vi "pulse_from memory tester.vi"() -> ()   [LabVIEW 2021]
uses:
  CTL/emitter params.ctl
  CTL/mode_type.ctl
  pdw.ctl
  <vilib>/addons/Modulation/Analog/controls/Complex Data Waveform.ctl
  <instrlib>/_niInstr/DSP/v1/Shared/Public/IQ Data.ctl
  <vilib>/addons/Modulation/Analog/support/Validators/mod_Fractional Resample Validate.vi
  <vilib>/addons/Modulation/Analog/support/Validators/mod_Check Flush State.vi
  <vilib>/addons/Modulation/Analog/support/mod_FractionalResampler.vi
  <vilib>/addons/Modulation/Analog/support/mod_Integer Rate Interpolation.vi
  <vilib>/addons/Modulation/Analog/support/mod_Set Error Source.vi
  <vilib>/addons/Modulation/Analog/support/Validators/mod_Validate Complex Waveform.vi
  <vilib>/addons/Modulation/Analog/support/mod_PerformResampling.vi
  <vilib>/addons/Modulation/Analog/support/Validators/mod_WFErrorHandler.vi
  <vilib>/sound2/lvsound2.llb/Sound File Read Open.vi
  <vilib>/sound2/lvsound2.llb/Sound File Read (DBL).vi
  <vilib>/Utility/error.llb/Error Cluster From Error Code.vi
  <vilib>/addons/Modulation/Analog/support/mod_Resampling Factors.vi
  <vilib>/addons/Modulation/Analog/support/mod_ResamplingFilter.vi
  <vilib>/addons/Modulation/Analog/support/mod_Generate Integer Interpolation Filter.vi
  <instrlib>/_niInstr/DSP/v1/FPGA/Public/Sub VIs/Data Conversion/IQ to U32 - 1 spc - S18.1.vi
  <vilib>/measure/maspectr.llb/FFT Power Spectrum and PSD for 1 Chan (CDB).vi
  <instrlib>/_niInstr/DSP/v1/FPGA/Public/Sub VIs/Data Conversion/U32 to IQ - N spc - S18.1.vi
  <vilib>/Analysis/NI_AALPro.lvlib
  <vilib>/measure/NI_MAPro.lvlib
  <instrlib>/_niInstr/Basic Elements/v1/FPGA/niInstr Basic Elements v1 FPGA.lvlib
  <vilib>/addons/Modulation/niAMT.lvlib
  <instrlib>/_niInstr/DSP/v1/Shared/niInstr DSP v1 Shared.lvlib
  <instrlib>/_niInstr/DSP/v1/FPGA/niInstr DSP v1 FPGA.lvlib
panel:
  in  "random bar":dbl
  out "start index":u16[](array[numeric])
  out "length":u16[](array[numeric])
  out "memory data":u32[](array[numeric])
  out "memory status 2":dbl[](graph)
  out "memory status":u32[](graph)
  out "Numeric":i32
  in  "num file":i32
  in  "IQ files":path[](array[path])=[path "C:/Users/PXIe8108_Demo/Documents/CHAIM DATA/chaim/5785_sync_for_elbit/tx_pulse/pulse Tx Folder_lv_21/EMEA_ADG_EW_Multi_Emitter_Scenarios/data/comb.wav"]
  out "D phase to Dt":dbl[](graph)
  out "output valid":i16[](graph)
  out "PDW in":T1={"PW"=60000, "frequency shift"=0.004999999999999005, "amp"=0.31623077392578125, "mode type"=enum."LFM", "mode depth"=234562481, "mode filter"=0, "phase shift"=0.0, "pulse shape filter"=0}
  out "free DDS":i16[](graph)
  out "Power Spectrum / PSD":cluster{"f0":dbl, "df":dbl, "magnitude":dbl[]}[](graph)
  out "amp out":dbl[](graph)
  out "phase out":dbl[](graph)
  in  "num of sampels for test":i32=30000 format="%.0p"
  out "I data":dbl[](graph)
  in  "emmiter":T3[](array[typedef])=[{"f set"=[1000000.0], "hop rate (Hz)"=1000.0, "d.c."=0.1, "amp (dB)"=-10.0, "mod type"=enum."from memory 1", "mod depth"=0.0, "DOA"=0.0, "t start"=0.0, "t end"=3.0}] {"t end" format="%#_3p"; "t start" format="%#_3p"; "DOA" format="%#_3p"; "mod depth" format="%.0p"}
  in  "Fs":i32=200000000 format="%#.3p"
  # "mode type:\n0- cw\n3-lfm\n4- bpsk\n5-qpsk"
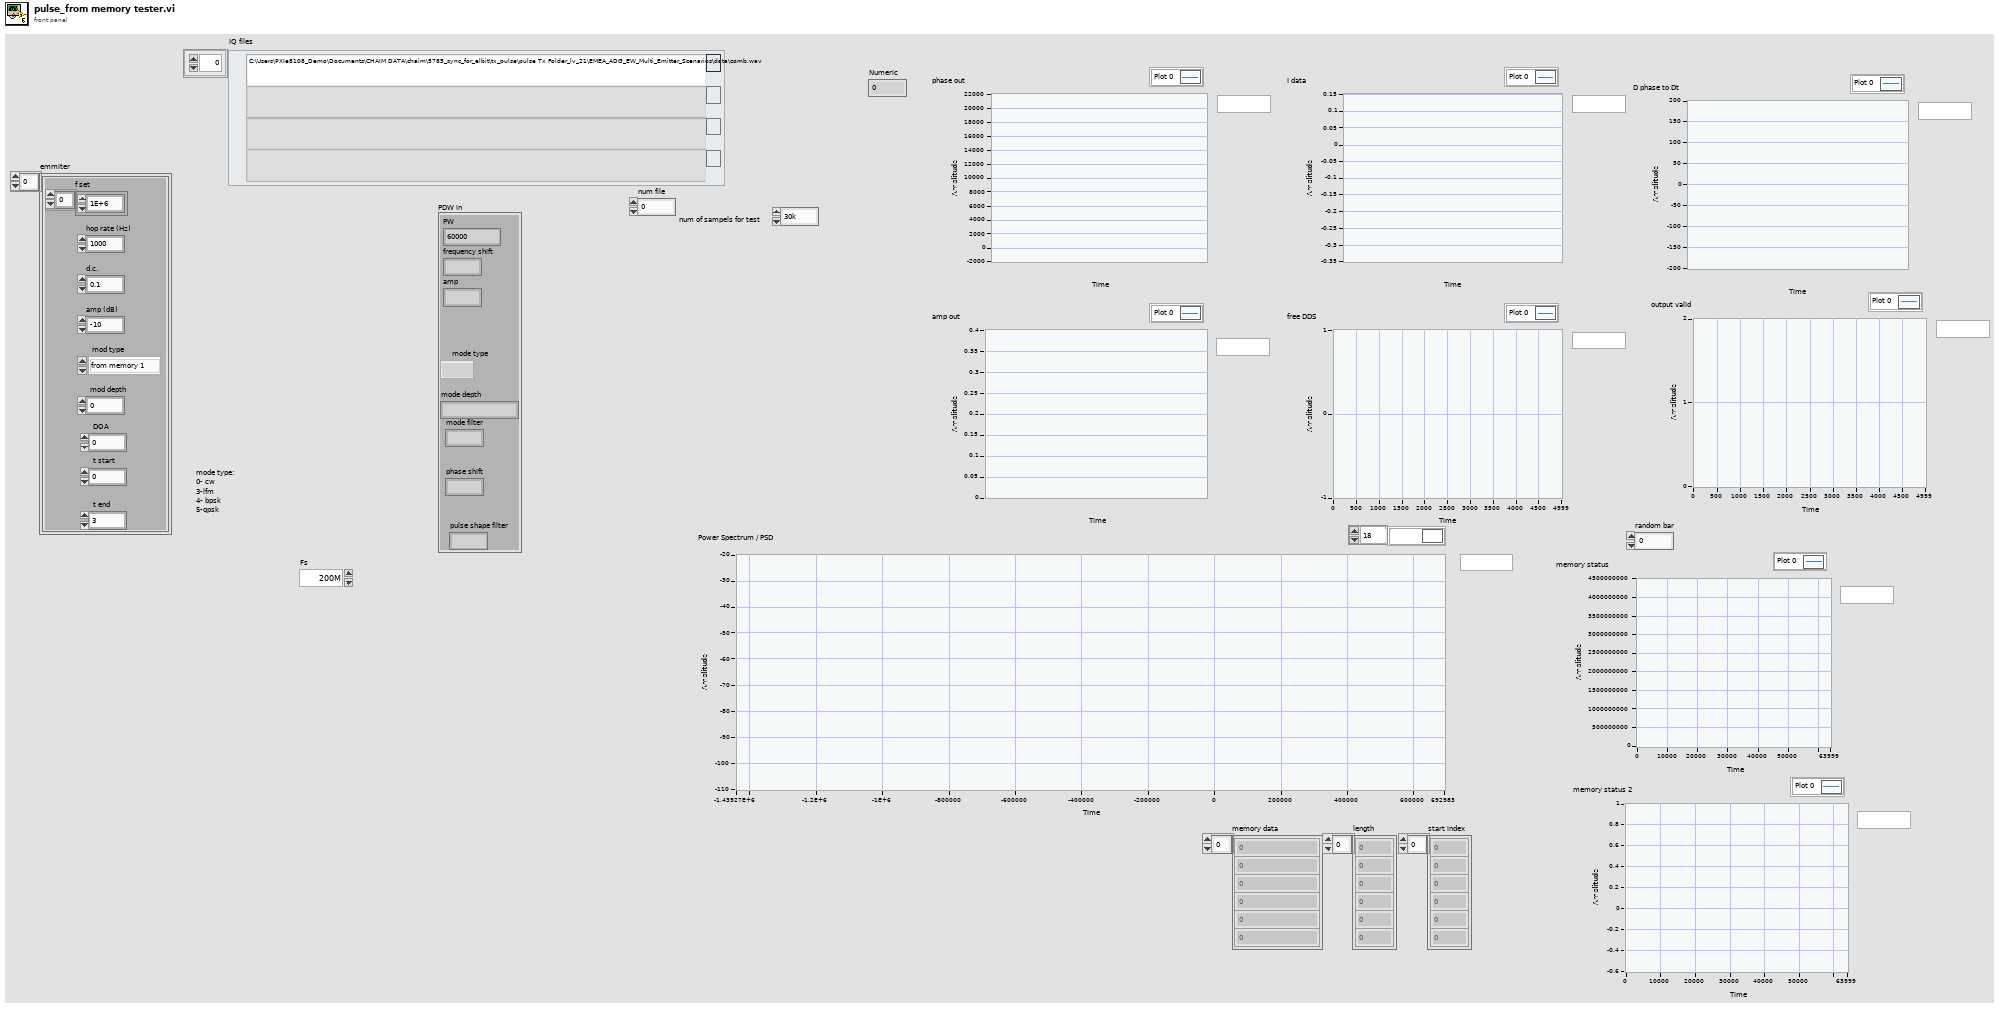
[diagram p1: front panel]
types:
  T1 = typedef "pdw.ctl" = cluster{"PW":u32, "frequency shift":fxp<+/-,48,0>, "amp":fxp<+/-,18,1>, "mode type":T2, "mode depth":u32, "mode filter":u8, "phase shift":fxp<+/-,16,1>, "pulse shape filter":u8}
  T2 = typedef "mode_type.ctl" = enum8{"CW", "from memory 1", "NC - cw", "LFM", "BPSK", "QPSK"}
  T3 = typedef "emitter params.ctl" = cluster{"f set":dbl[], "hop rate (Hz)":dbl, "d.c.":dbl, "amp (dB)":dbl, "mod type":T2, "mod depth":dbl, "DOA":dbl, "t start":dbl, "t end":dbl}
  T4 = typedef "niAMT.lvlib/Complex Data Waveform.ctl" = cluster{"t0":dbl, "dt":dbl, "Y":cdb[]}
  T5 = typedef "niInstr DSP v1 Shared.lvlib/IQ Data.ctl" = cluster{"I":fxp<+/-,18,1>, "Q":fxp<+/-,18,1>, "overflow":bool}
  T6 = typedef "Sound File Refnum.ctl" = refnum<file>
  T7 = typedef "PDW_lv2.ctl" = cluster{"t start":dbl, "frequency (Hz)":dbl, "duration (sec)":dbl, "mod type":T2, "mod depth":dbl, "phase (rad)":dbl[], "amp (lin)":dbl[]}
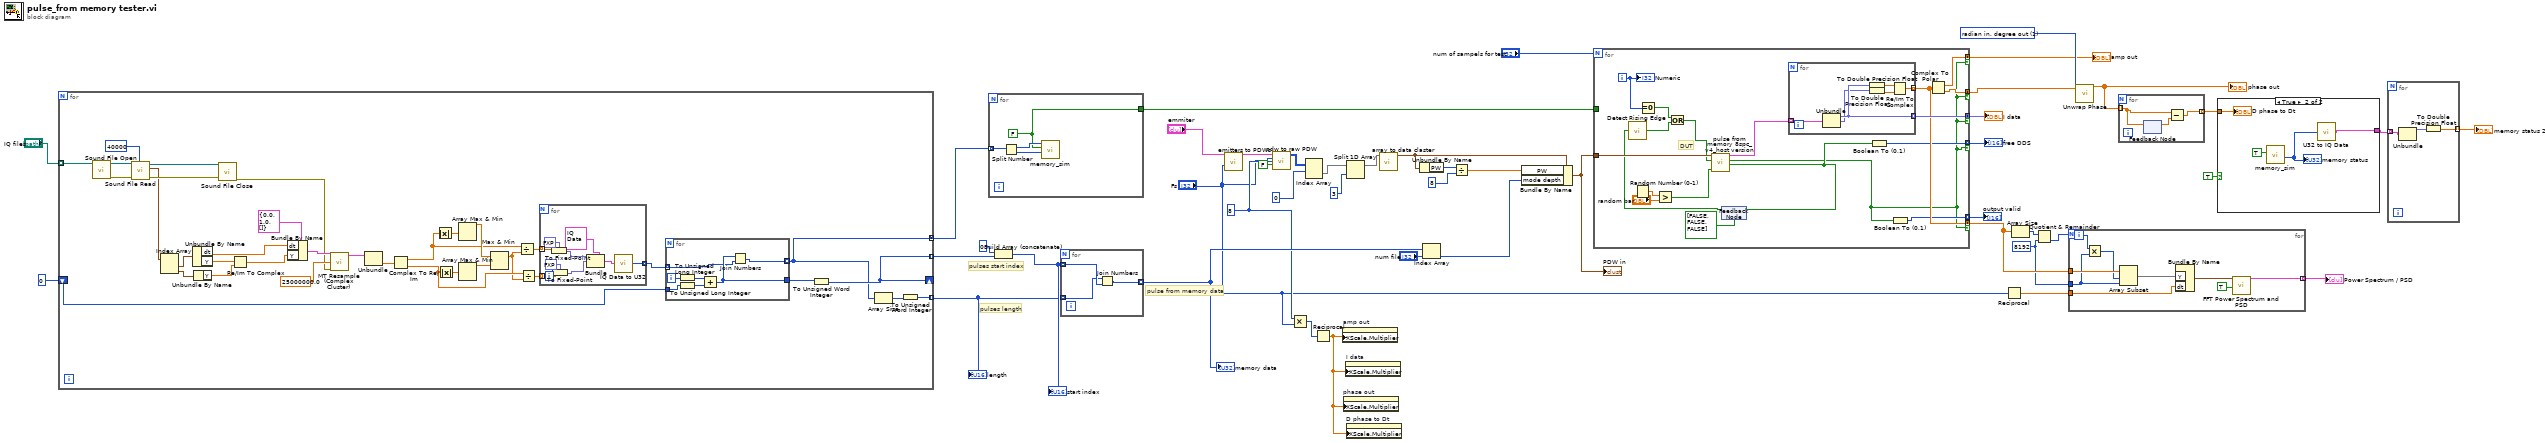
[diagram p0: block diagram]
diagram:
  w4 = 8 ("SPC")
  w35 = 8192 ("length")
  w44 = 1 items=["radian in, radian out", "radian in, degree out", "degree in, degree out", "degree in, radian out"] ("phase unit")
  # "pulse from memory data"
  # "pulses start index"
  # "pulses length"
  n1 = for {
    shift-right: [w53] -> _
    shift-left: u16 0 -> [w55]
    tunnel: [w48] -> w18 mode=concatenating
    tunnel: [w51] -> w20 mode=indexing
    tunnel: [w53] -> w19 mode=indexing
    tunnel: "IQ files" -> [w50] mode=indexing
    n2 = call-poly <vilib>:"Sound File Open.vi"("path"=w50) -> ("error out"=w78:errorcluster, "sound file refnum"=w81:T6)  [unwired: 9 in]
    n3 = call-poly <vilib>:"Sound File Read.vi"("number of samples/ch (-1: all)"=40000, "error in (no error)"=w78, "sound file refnum"=w81) -> ("error out"=w77:errorcluster, "data"=w76:waveform(dbl)[], "sound file refnum out"=w80:T6)  [unwired: 4 in, 2 out]
    n4 = Index Array(array=w76) -> (element #1=w75:waveform(dbl), element #2=w74:waveform(dbl))  [unwired: 2 in]
    n5 = Unbundle By Name(w75) -> ("dt"=w70:dbl, "Y"=w73:dbl[])
    n6 = Unbundle By Name(w74) -> ("Y"=w72:dbl[])
    n7 = call <vilib>:"Sound File Close.vi"("error in (no error)"=w77, "sound file refnum"=w80) -> ("error out"=w60:errorcluster)  [unwired: 9 in]
    n8 = Re/Im To Complex(1:w72, 2:w73) -> (0:w69:cdb[])
    n9 = Bundle By Name(cluster=T4 {"t0"=0.0, "dt"=1.0, "Y"=[]} ("input complex waveform"), "dt"=w70, "Y"=w69) -> (w68:T4)
    n10 = call <vilib>:"MT Resample (Complex Cluster).vi"("input complex waveform"=w68, "desired sample rate (Hz)"=25000000.0, "error in (no error)"=w60) -> ("output complex waveform"=w58:T4)  [unwired: 11 in, 1 out]
    n11 = Unbundle(w58) -> ("Y"=w66:cdb[])  [unwired: 2 out]
    n12 = Complex To Re/Im(x + iy=w66) -> (x=w49:dbl[], y=w61:dbl[])
    n13 = Absolute Value(x=w49) -> (abs(x)=w63:dbl[])
    n14 = Absolute Value(x=w61) -> (abs(x)=w62:dbl[])
    n15 = Array Max & Min(array=w63) -> (max value=w64:dbl)  [unwired: 3 out]
    n16 = Array Max & Min(array=w62) -> (max value=w65:dbl)  [unwired: 3 out]
    n17 = Max & Min(x=w64, y=w65) -> (max(x,y)=w59:dbl)  [unwired: 1 out]
    n18 = Divide(x=w49, y=w59) -> (x/y=w57:dbl[])
    n19 = Divide(x=w61, y=w59) -> (x/y=w47:dbl[])
    n20 = for {
      tunnel: w47 -> [w88] mode=indexing
      tunnel: w57 -> [w85] mode=indexing
      tunnel: [w82] -> w56 mode=indexing
      n21 = To Fixed-Point(fixed-point type=fxp<+/-,18,1> 0.0 ("I"), number=w85) -> (fixed-point=w84:fxp<+/-,18,1>)
      n22 = To Fixed-Point(fixed-point type=fxp<+/-,18,1> 0.0 ("I"), number=w88) -> (fixed-point=w89:fxp<+/-,18,1>)
      n23 = Bundle(cluster=T5 {"I"=0.0, "Q"=0.0, "overflow"=FALSE} ("IQ data"), "I"=w84, "Q"=w89) -> (w83:T5)  [unwired: 1 in]
      n24 = call-poly <instrlib>:"IQ Data to U32.vi"("IQ data"=w83) -> ("U32 data"=w82:u32)  [unwired: 13 in, 1 out]
    }
    n25 = for {
      tunnel: [w97] -> w48 mode=indexing
      tunnel: [w96] -> w54
      tunnel: w55 -> [w92]
      tunnel: w56 -> [w95] mode=indexing
      i -> [w94]
      n26 = To Unsigned Long Integer(number=w94) -> (unsigned 32bit integer=w93:u32)
      n27 = To Unsigned Long Integer(number=w92) -> (unsigned 32bit integer=w91:u32)
      n28 = Add(x=w93, y=w91) -> (x+y=w96:u32)
      n29 = Join Numbers(hi=w96, lo=w95) -> ((hi.lo)=w97:u64)
    }
    n30 = To Unsigned Word Integer(number=w54) -> (unsigned 16bit integer=w53:u16)
    n31 = Array Size(array=w48) -> (size(s)=w52:i32)
    n32 = To Unsigned Word Integer(number=w52) -> (unsigned 16bit integer=w51:u16)
  }
  "length" <- w20
  n33 = for {
    tunnel: w18 -> [w101] mode=indexing
    tunnel: [w98] -> w1
    w98 = FALSE ("t-read;fwrite")
    n34 = Split Number(x=w101) -> (hi(x)=w100:u32, lo(x)=w99:u32)
    n35 = call "memory_sim.vi"("data in"=w99, "t-read;fwrite"=w98, "index"=w100) -> ()  [unwired: 7 in, 2 out]
  }
  n36 = Build Array (concatenate)(u16 0, w19) -> (w22:u16[])
  "start index" <- w22
  n37 = for {
    tunnel: w22 -> [w104] mode=indexing
    tunnel: w20 -> [w103] mode=indexing
    tunnel: [w102] -> w17 mode=indexing
    n38 = Join Numbers(hi=w103, lo=w104) -> ((hi.lo)=w102:u32)
  }
  "memory data" <- w17
  n39 = call "emitters to PDWs.vi"("emmiter"="emmiter", "center frequency (Hz)"="Fs") -> ("sorted array"=w41:T7[])  [unwired: 11 in, 2 out]
  n40 = call "pdw to raw PDW.vi"("PDWs"=w41, "Fs fpGa"="Fs", "SPC"=w4, "gen for DF"=FALSE) -> ("Array"=w29:u64[][])  [unwired: 9 in, 2 out]
  n41 = Multiply(x=w4, y="Fs") -> (x*y=w2:i32)
  n42 = Index Array(array=w29, index (row)=0) -> (element=w26:u64[])  [unwired: 1 in]
  n43 = Reciprocal(x=w2) -> (1/x=w5:dbl)
  n44 = property on="amp out" class="WFGraph (strict)"("XScale.Multiplier"=w5) -> ()  [unwired: 2 in, 2 out]
  n45 = property on="phase out" class="WFGraph (strict)"("XScale.Multiplier"=w5) -> ()  [unwired: 2 in, 2 out]
  n46 = property on="I data" class="WFGraph (strict)"("XScale.Multiplier"=w5) -> ()  [unwired: 2 in, 2 out]
  n47 = property on="D phase to Dt" class="WFGraph (strict)"("XScale.Multiplier"=w5) -> ()  [unwired: 2 in, 2 out]
  n48 = Split 1D Array(array=w26, index=3) -> (first subarray=w24:u64[])  [unwired: 1 out]
  n49 = call "array to data claster.vi"("Array"=w24) -> ("Cluster"=w9:T1)  [unwired: 10 in]
  n50 = Unbundle By Name(w9) -> ("PW"=w8:u32)
  n51 = Index Array(array=w17, index="num file") -> (element=w15:u32)
  n52 = Divide(x=w8, y=u32 8) -> (x/y=w6:dbl)
  n53 = Bundle By Name(cluster=w9, "PW"=w6, "mode depth"=w15) -> (w10:T1)
  "PDW in" <- w10
  n54 = for {
    N: "num of sampels for test" -> [_]
    tunnel: [w122] -> w46 mode=concatenating if=w110
    tunnel: [w119] -> w45 mode=concatenating if=w110
    tunnel: [w120] -> w43 mode=concatenating if=w110
    tunnel: w10 -> [w121]
    tunnel: [w118] -> w39 mode=concatenating if=w110
    tunnel: [w117] -> w37 mode=indexing if=w110
    tunnel: [w116] -> w32 mode=indexing
    tunnel: w1 -> [_]
    i -> [w108]
    # "DUT"
    n55 = Random Number (0-1)() -> (number: 0 to 1=w113:dbl)
    n56 = Equal To 0?(x=w108) -> (x = 0?=w107:bool)
    n57 = Greater?(x=w113, y="random bar") -> (0:w111:bool)
    n58 = feedback #1(bool[] [FALSE, FALSE, FALSE]) -> (w115:bool)
    n59 = call <instrlib>:"Detect Rising Edge.vi"("signal"=w115) -> ("edge detected"=w106:bool)  [unwired: 14 in]
    n60 = Or(x=w107, y=w106) -> (x .or. y?=w105:bool)
    n61 = call "pulse from memory 8spc_v4_host version.vi"("run"=w111, "start this pulse"=w105, "PDW"=w121) -> ("free DDS"=w114:bool, "output valid"=w110:bool, "IQ_out"=w123:T5[])  [unwired: 6 in]
    n62 = feedback-in #1(w114) -> ()
    n63 = for {
      tunnel: w123 -> [w129] mode=indexing
      tunnel: [w128] -> w122 mode=indexing
      tunnel: [w126] -> w118 mode=indexing
      n64 = Unbundle(w129) -> ("I"=w128:fxp<+/-,18,1>, "Q"=w127:fxp<+/-,18,1>)  [unwired: 1 out]
      n65 = To Double Precision Float(number=w128) -> (double precision float=w125:dbl)
      n66 = To Double Precision Float(number=w127) -> (double precision float=w124:dbl)
      n67 = Re/Im To Complex(1:w124, 2:w125) -> (0:w126:cdb)
    }
    n68 = Boolean To (0,1)(Boolean=w114) -> (0, 1=w117:i16)
    n69 = Boolean To (0,1)(Boolean=w110) -> (0, 1=w116:i16)
    n70 = Complex To Polar(r * e^(i*theta)=w118) -> (r=w120:dbl[], theta=w119:dbl[])
    "Numeric" <- w108
  }
  "I data" <- w46
  "amp out" <- w43
  "free DDS" <- w37
  "output valid" <- w32
  n71 = Reciprocal(x="Fs") -> (1/x=w40:dbl)
  n72 = Array Size(array=w39) -> (size(s)=w36:i32)
  n73 = Quotient & Remainder(x=w36, y=w35) -> (floor(x/y)=w34:i32)  [unwired: 1 out]
  n74 = for {
    N: w34 -> [_]
    tunnel: w39 -> [w135]
    tunnel: w40 -> [w134]
    tunnel: w35 -> [w133]
    tunnel: [w131] -> w33 mode=indexing
    i -> [w130]
    n75 = Multiply(x=w130, y=w133) -> (x*y=w132:i32)
    n76 = Array Subset(array=w135, index=w132, length=w133) -> (w136:cdb[])
    n77 = Bundle By Name("Y"=w136, "dt"=w134) -> (w138:waveform(cdb))  [unwired: 1 in]
    n78 = call-poly <vilib>:"FFT Power Spectrum and PSD.vi"("dB On (F)"=TRUE, "time signal"=w138) -> ("Power Spectrum / PSD"=w131:cluster{"f0":dbl, "df":dbl, "magnitude":dbl[]})  [unwired: 6 in, 3 out]
  }
  "Power Spectrum / PSD" <- w33
  n79 = call <vilib>:"Unwrap Phase.vi"("phase unit"=w44, "Phase"=w45) -> ("Unwrapped Phase"=w31:dbl[])  [unwired: 8 in, 1 out]
  "phase out" <- w31
  n80 = for {
    tunnel: w31 -> [w141] mode=indexing
    tunnel: [w139] -> w30 mode=indexing
    n81 = feedback-in #2(w141) -> ()
    n82 = feedback #2() -> (w140:dbl)  [unwired: 1 in]
    n83 = Subtract(x=w141, y=w140) -> (x-y=w139:dbl)
  }
  n84 = case shown="True" TRUE {
    tunnel: w30 -> [_ w145]
    tunnel: [_ w143] -> w12
    frame False {
    }
    frame True {
      n85 = call "memory_sim.vi"("t-read;fwrite"=TRUE) -> ("Array"=w144:u32[])  [unwired: 9 in, 1 out]
      "memory status" <- w144
      n86 = call-poly <instrlib>:"U32 to IQ Data.vi"("U32 data"=w144) -> ("IQ data"=w143:T5[])  [unwired: 14 in]
      "D phase to Dt" <- w145
    }
  }
  n87 = for {
    tunnel: w12 -> [w148] mode=indexing
    tunnel: [w146] -> w11 mode=indexing
    n88 = Unbundle(w148) -> ("I"=w147:fxp<+/-,18,1>)  [unwired: 2 out]
    n89 = To Double Precision Float(number=w147) -> (double precision float=w146:dbl)
  }
  "memory status 2" <- w11
